vi "DataFileCreator_MR.vi"(10 "ProjectName":string="QFinger", 11 "Folder path input":path=path "C:/Labview34970A stuff/Data") -> (2 "NewFileCreated":string, 3 "NewFilePath":path)   [LabVIEW 2016]
doc: "Given an input Folder path this VI creates the next data file in the format \n2017-09-17ProjectName#001\nIt only checks the latest file in the folder to decide if a sequence with today's date already exists.\nIf the file sequence has not been started, it creates one begining with #001\nIf it happens that it tries to create a file that already exists, a dialog pops up\nasking for a new name."
panel:
  out "filenames":string[](array[string])
  out "Newest file containing a #+3chars":string
  out "end of newest file name":string
  out "File time stamps sorted by time":timestamp[](array[timestamp])
  out "Files in Folder sorted by time":path[](array[path])
  out "FileTypeExists?":bool
  out "date string":string
  out "DayParsed":string
  out "MonthParsed":string
  out "YearParsed":string
  out "newest existing file":string
  # "Given an input Folder path this VI creates the next data file in the format \n2017-09-17ProjectName#001\nIt only checks the latest file in the folder to decide if \na sequence with today's date already exists.\nIf the file sequence has not been started, it creates one begining with #001\nIf it happens that it tries to create a file that already exists, a dialog pops up\nasking for a new name.\n2017 11 07- now this finds the newest file containing a # so it doesn't get confused if\nthere is a log file that is newer than the latest data file"
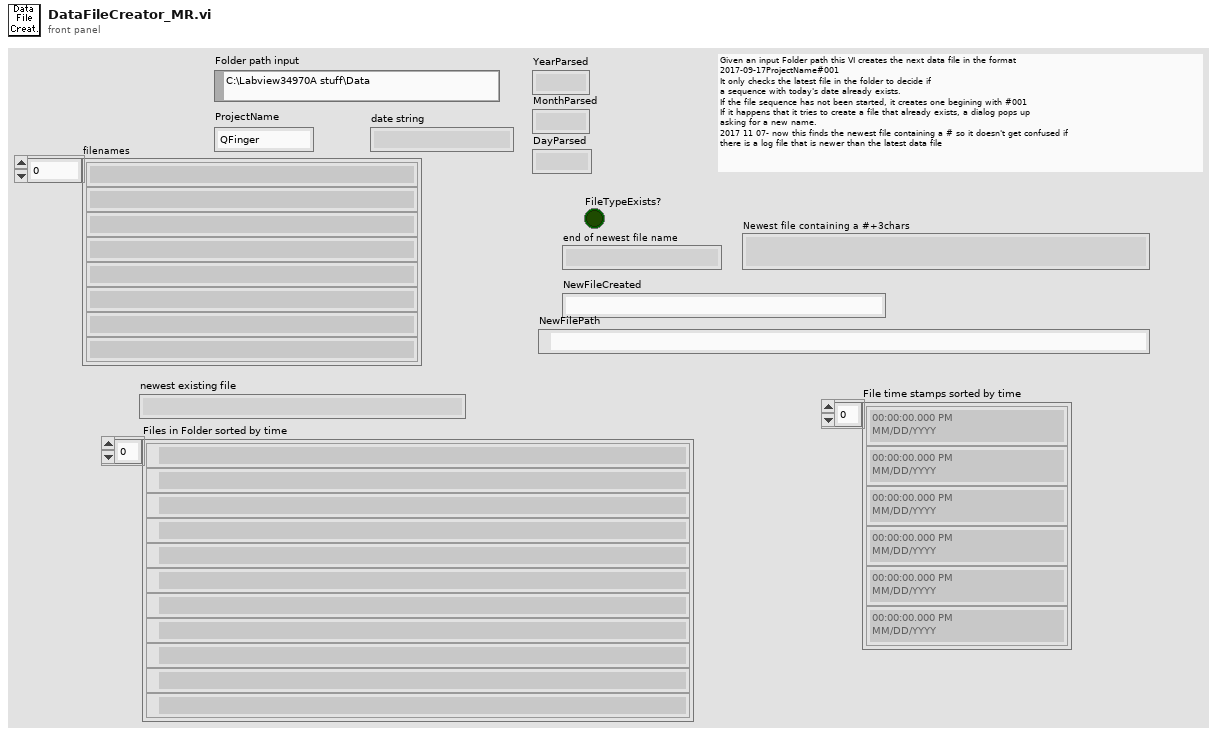
[diagram p1: front panel]
types:
  T1 = enum16{"open", "replace", "create", "open or create", "replace or create", "replace or create with confirmation"}
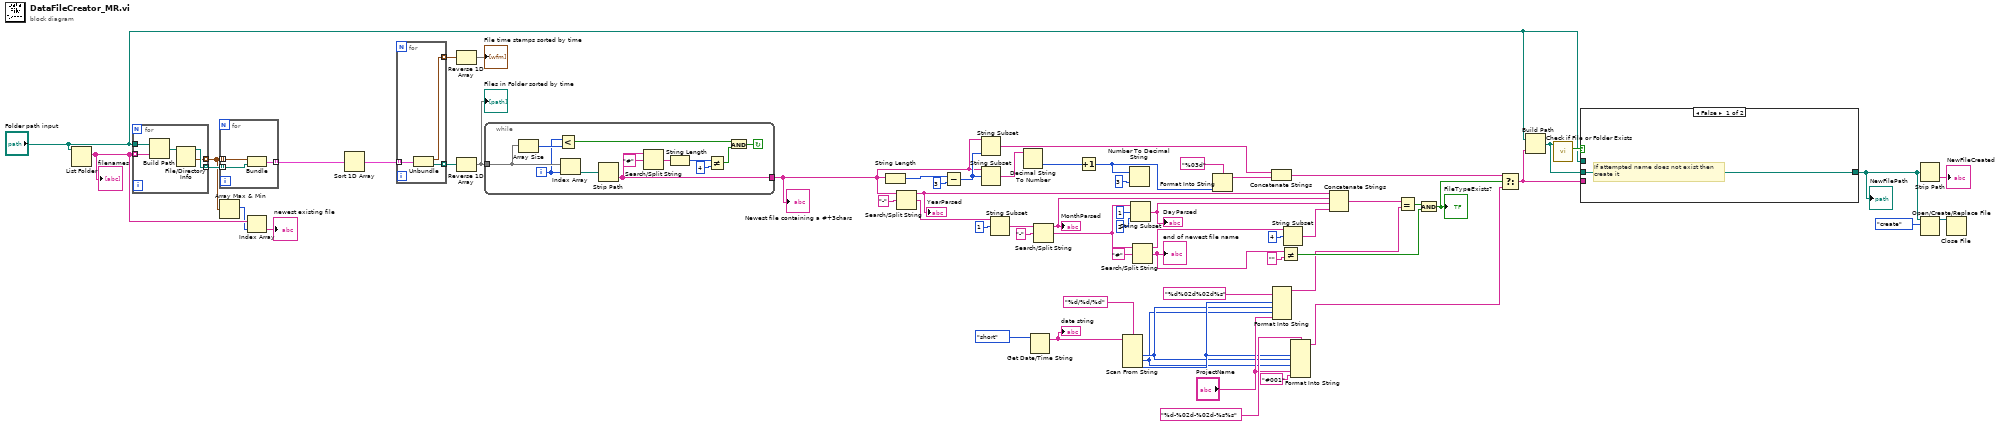
[diagram p0: block diagram]
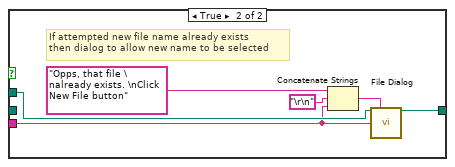
[diagram p2: hidden frame]
diagram:
  n1 = List Folder(path="Folder path input") -> (filenames=w17:string[])  [unwired: 3 in, 3 out]
  "filenames" <- w17
  n2 = for {
    tunnel: w17 -> [w69] mode=indexing
    tunnel: [w67] -> w29 mode=indexing
    tunnel: [w66] -> w28 mode=indexing
    tunnel: "Folder path input" -> [w65]
    n3 = Build Path(base path=w65, name or relative path=w69) -> (appended path=w68:path)
    n4 = File/Directory Info(path=w68) -> (path out=w67:path, last mod=w66:timestamp)  [unwired: 1 in, 5 out]
  }
  n5 = for {
    tunnel: w28 -> [w72] mode=indexing
    tunnel: w29 -> [w71] mode=indexing
    tunnel: [w70] -> w33 mode=indexing
    n6 = Bundle("last mod"=w72, "path out"=w71) -> (w70:cluster{"last mod":timestamp, "path out":path})  [unwired: 1 in]
  }
  n7 = Array Max & Min(array=w28) -> (max index (indices)=w16:i32)  [unwired: 3 out]
  n8 = Index Array(array=w17, index=w16) -> (element=→"newest existing file":string)
  n9 = Sort 1D Array(array=w33) -> (sorted array=w32:cluster{"last mod":timestamp, "path out":path}[])
  n10 = for {
    tunnel: w32 -> [w75] mode=indexing
    tunnel: [w74] -> w15 mode=indexing
    tunnel: [w73] -> w31 mode=indexing
    n11 = Unbundle(w75) -> ("last mod"=w73:timestamp, "path out"=w74:path)
  }
  n12 = Reverse 1D Array(array=w31) -> (reversed array=→"File time stamps sorted by time":timestamp[])
  n13 = Reverse 1D Array(array=w15) -> (reversed array=w14:path[])
  "Files in Folder sorted by time" <- w14
  n14 = while {
    tunnel: w14 -> [w85]
    tunnel: [w80] -> w13
    i -> [w83]
    stop <- w86 continue-if-true
    n15 = Array Size(array=w85) -> (size(s)=w84:i32)
    n16 = Less?(x=w83, y=w84) -> (x < y?=w82:bool)
    n17 = Index Array(array=w85, index=w83) -> (element=w81:path)
    n18 = Strip Path(path=w81) -> (name=w80:string)  [unwired: 1 out]
    n19 = Search/Split String(string=w80, search string/char (-)="#") -> (match + rest of string=w79:string)  [unwired: 1 in, 2 out]
    n20 = String Length(string=w79) -> (length=w78:i32)
    n21 = Not Equal?(x=w78, y=4) -> (x != y?=w76:bool)
    n22 = And(x=w82, y=w76) -> (x .and. y?=w86:bool)
  }
  "Newest file containing a #+3chars" <- w13
  n23 = String Length(string=w13) -> (length=w50:i32)
  n24 = Search/Split String(string=w13, search string/char (-)="-") -> (substring before match=w52:string, match + rest of string=w61:string)  [unwired: 1 in, 1 out]
  "YearParsed" <- w52
  n25 = Subtract(x=w50, y=3) -> (x-y=w48:i32)
  n26 = String Subset(string=w13, length (rest)=w48) -> (substring=w42:string)  [unwired: 1 in]
  n27 = String Subset(string=w13, offset (0)=w48) -> (substring=w47:string)  [unwired: 1 in]
  n28 = String Subset(string=w61, offset (0)=1) -> (substring=w60:string)  [unwired: 1 in]
  n29 = Decimal String To Number(string=w47) -> (number=w46:i32)  [unwired: 2 in, 1 out]
  n30 = Get Date/Time String(date format (0)=enum16{"short", "long", "abbreviated"}."short") -> (date string=w10:string)  [unwired: 2 in, 1 out]
  "date string" <- w10
  n31 = Search/Split String(string=w60, search string/char (-)="-") -> (substring before match=w56:string, match + rest of string=w25:string)  [unwired: 1 in, 1 out]
  "MonthParsed" <- w56
  n32 = Increment(x=w46) -> (x+1=w44:i32)
  n33 = Scan From String(format string="%d/%d/%d", input string=w10) -> (output 1=w2:i32, output 2=w1:i32, output 3=w3:i32)  [unwired: 5 in, 3 out]
  n34 = Number To Decimal String(number=w44, width (-)=i16 3) -> ()  [unwired: 1 out]
  n35 = String Subset(string=w25, offset (0)=1, length (rest)=2 ("y")) -> (substring=w55:string)
  "DayParsed" <- w55
  n36 = Search/Split String(string=w25, search string/char (-)="#") -> (substring before match=w24:string, match + rest of string=w22:string)  [unwired: 1 in, 1 out]
  "end of newest file name" <- w22
  n37 = Format Into String(format string="%03d", w44) -> (resulting string=w41:string)  [unwired: 2 in, 1 out]
  n38 = Concatenate Strings(w42, w41) -> (w51:string)
  n39 = Format Into String(format string="%d%02d%02d%s", w3, w2, w1, "ProjectName") -> (resulting string=w5:string)  [unwired: 2 in, 1 out]
  n40 = Not Equal?(x=w22, y="") -> (x != y?=w20:bool)
  n41 = String Subset(string=w24, offset (0)=4) -> (substring=w23:string)  [unwired: 1 in]
  n42 = Format Into String(format string="%d-%02d-%02d-%s%s", w3, w2, w1, "ProjectName", "#001" ("string")) -> (resulting string=w4:string)  [unwired: 2 in, 1 out]
  n43 = Concatenate Strings(w52, w56, w55, w23) -> (w54:string)
  n44 = Equal?(x=w54, y=w5) -> (x = y?=w19:bool)
  n45 = And(x=w19, y=w20) -> (x .and. y?=w18:bool)
  "FileTypeExists?" <- w18
  n46 = Select(t=w51, s=w18, f=w4) -> (s? t:f=w36:string)
  n47 = Build Path(base path="Folder path input", name or relative path=w36) -> (appended path=w40:path)
  n48 = call <vilib>:"Check if File or Folder Exists.vi"("path"=w40) -> ("file or folder exists?"=w39:bool)  [unwired: 8 in, 2 out]
  n49 = case shown="False" w39 {
    tunnel: w40 -> [w88 _]
    tunnel: "Folder path input" -> [_ w94]
    tunnel: [w88 w93] -> w34
    tunnel: w36 -> [_ w89]
    frame False {
      # "If attempted name does not exist then \ncreate it"
    }
    frame True {
      # "If attempted new file name already exists\nthen dialog to allow new name to be selected"
      n50 = Concatenate Strings("Opps, that file \nalready exists. \nClick New File button" ("prompt"), "\r\n", w89) -> (w90:string)
      n51 = call "File Dialog"("start path"=w94, "prompt"=w90, "default name"=w89) -> ("selected path"=w93:path)  [unwired: 9 in, 3 out]
    }
  }
  "NewFilePath" <- w34
  n52 = Strip Path(path=w34) -> (name=→"NewFileCreated":string)  [unwired: 1 out]
  n53 = Open/Create/Replace File(file path (use dialog)=w34, operation (0:open)=T1."create") -> (refnum out=w37:refnum<file>)  [unwired: 4 in, 2 out]
  n54 = Close File(refnum=w37) -> ()  [unwired: 1 in, 2 out]
